vi "tests.vi"   [LabVIEW 2018]
uses:
  RxTx/RxTx.lvclass
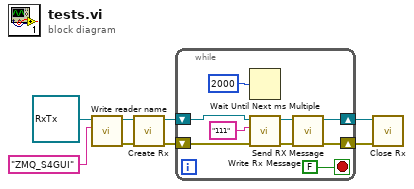
[diagram p0: block diagram]
diagram:
  n1 = call-dynamic "Write reader name.vi"("RX name"="ZMQ_S4GUI", "RxTx in"=refnum<class "RxTx.lvclass"> refnum) -> ("error out"=w3:errorcluster, "RxTx out"=w4:refnum<class "RxTx.lvclass">)  [unwired: 8 in]
  n2 = call "Create Rx.vi"("error in (no error)"=w3, "RxTx in"=w4) -> ("error out"=w5:errorcluster, "RxTx out"=w8:refnum<class "RxTx.lvclass">)  [unwired: 8 in]
  n3 = while {
    shift-right: [w15] -> w7
    shift-left: w8 -> [w17]
    shift-right: [w14] -> w6
    shift-left: w5 -> [w12]
    stop <- FALSE stop-if-true
    n4 = Wait Until Next ms Multiple(millisecond multiple=u32 2000) -> ()  [unwired: 1 out]
    n5 = call "Write Rx Message.vi"("error in (no error)"=w12, "Rx Message"="111", "RxTx in"=w17) -> ("error out"=w13:errorcluster, "RxTx out"=w16:refnum<class "RxTx.lvclass">)  [unwired: 7 in]
    n6 = call "Send RX Message.vi"("error in (no error)"=w13, "RxTx in"=w16) -> ("error out"=w14:errorcluster, "RxTx out"=w15:refnum<class "RxTx.lvclass">)  [unwired: 8 in]
  }
  n7 = call "Close Rx.vi"("error in (no error)"=w6, "RxTx in"=w7) -> ()  [unwired: 8 in, 2 out]
